vi "Build Channel List.vi"(9 "Channel":u32, 10 "Data line":u16, 11 "Protocol capture resource name":string) -> (3 "String":string)   [LabVIEW 2021, in "audio adc shared.lvlib"]
uses:
  audio adc shared.lvlib
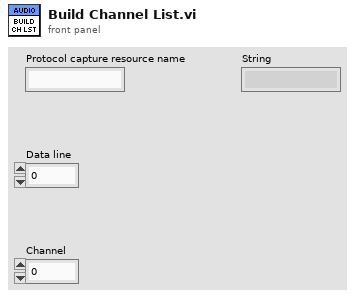
[diagram p1: front panel]
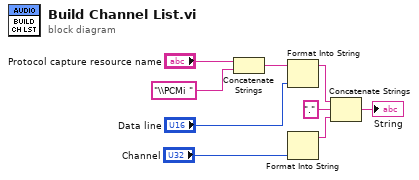
[diagram p0: block diagram]
diagram:
  n1 = Concatenate Strings("Protocol capture resource name", "\\PCMi " ("string")) -> (w1:string)
  n2 = Format Into String(initial string=w1, "Data line") -> (resulting string=w6:string)  [unwired: 2 in, 1 out]
  n3 = Format Into String("Channel") -> (resulting string=w8:string)  [unwired: 3 in, 1 out]
  n4 = Concatenate Strings(w6, "." ("string"), w8) -> (→"String":string)
